vi "DAQ@AddDAQ__Parameter.vi"(1 "ParamterIn":string) -> (0 "ParamterOut":string)   [LabVIEW 2020]
uses:
  MainFrame/Global.vi
panel:
  out "Example Setting:":string
  in  "Dev=":string(combo)
  in  "INTYPE=":string(combo)
  in  "Vmin=":string(combo)
  in  "Vmax=":string(combo)
  in  "Len=":string(combo)
  in  "SPS=":string(combo)
  in  "Ch=":string(combo)
  in  "Driver":string(combo)
  in  "DAQName":string(combo)
  in  "Confirm":bool
  # "Name"
  # "Driver"
  # "Device"
  # "Channel"
  # "Samples Per Second"
  # "SPS"
  # "Range"
  # "~"
  # "Data\nLength"
  # "Second"
  # "Type"
  # "$NAME,NIDAQAI,DEV=,CH=0:1,SPS=,RANGE=-5~5,LEN=,INTYPE=\n$NAME,NIDAQAO,DEV=,CH=0:1,SPS=,RANGE=-5~5"
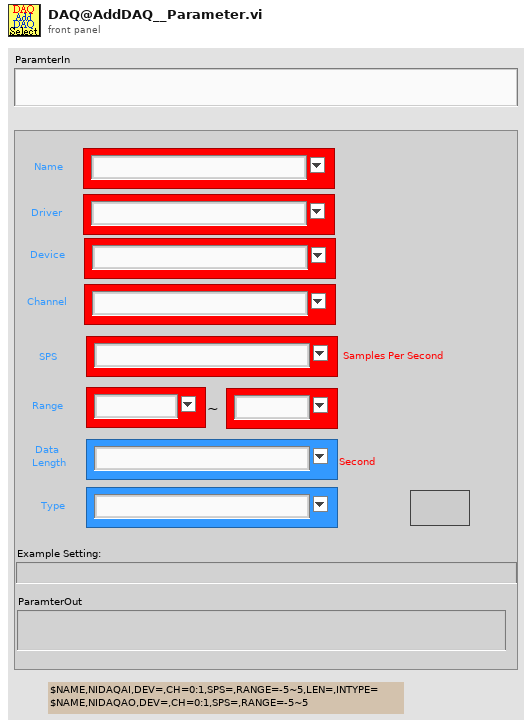
[diagram p1: front panel]
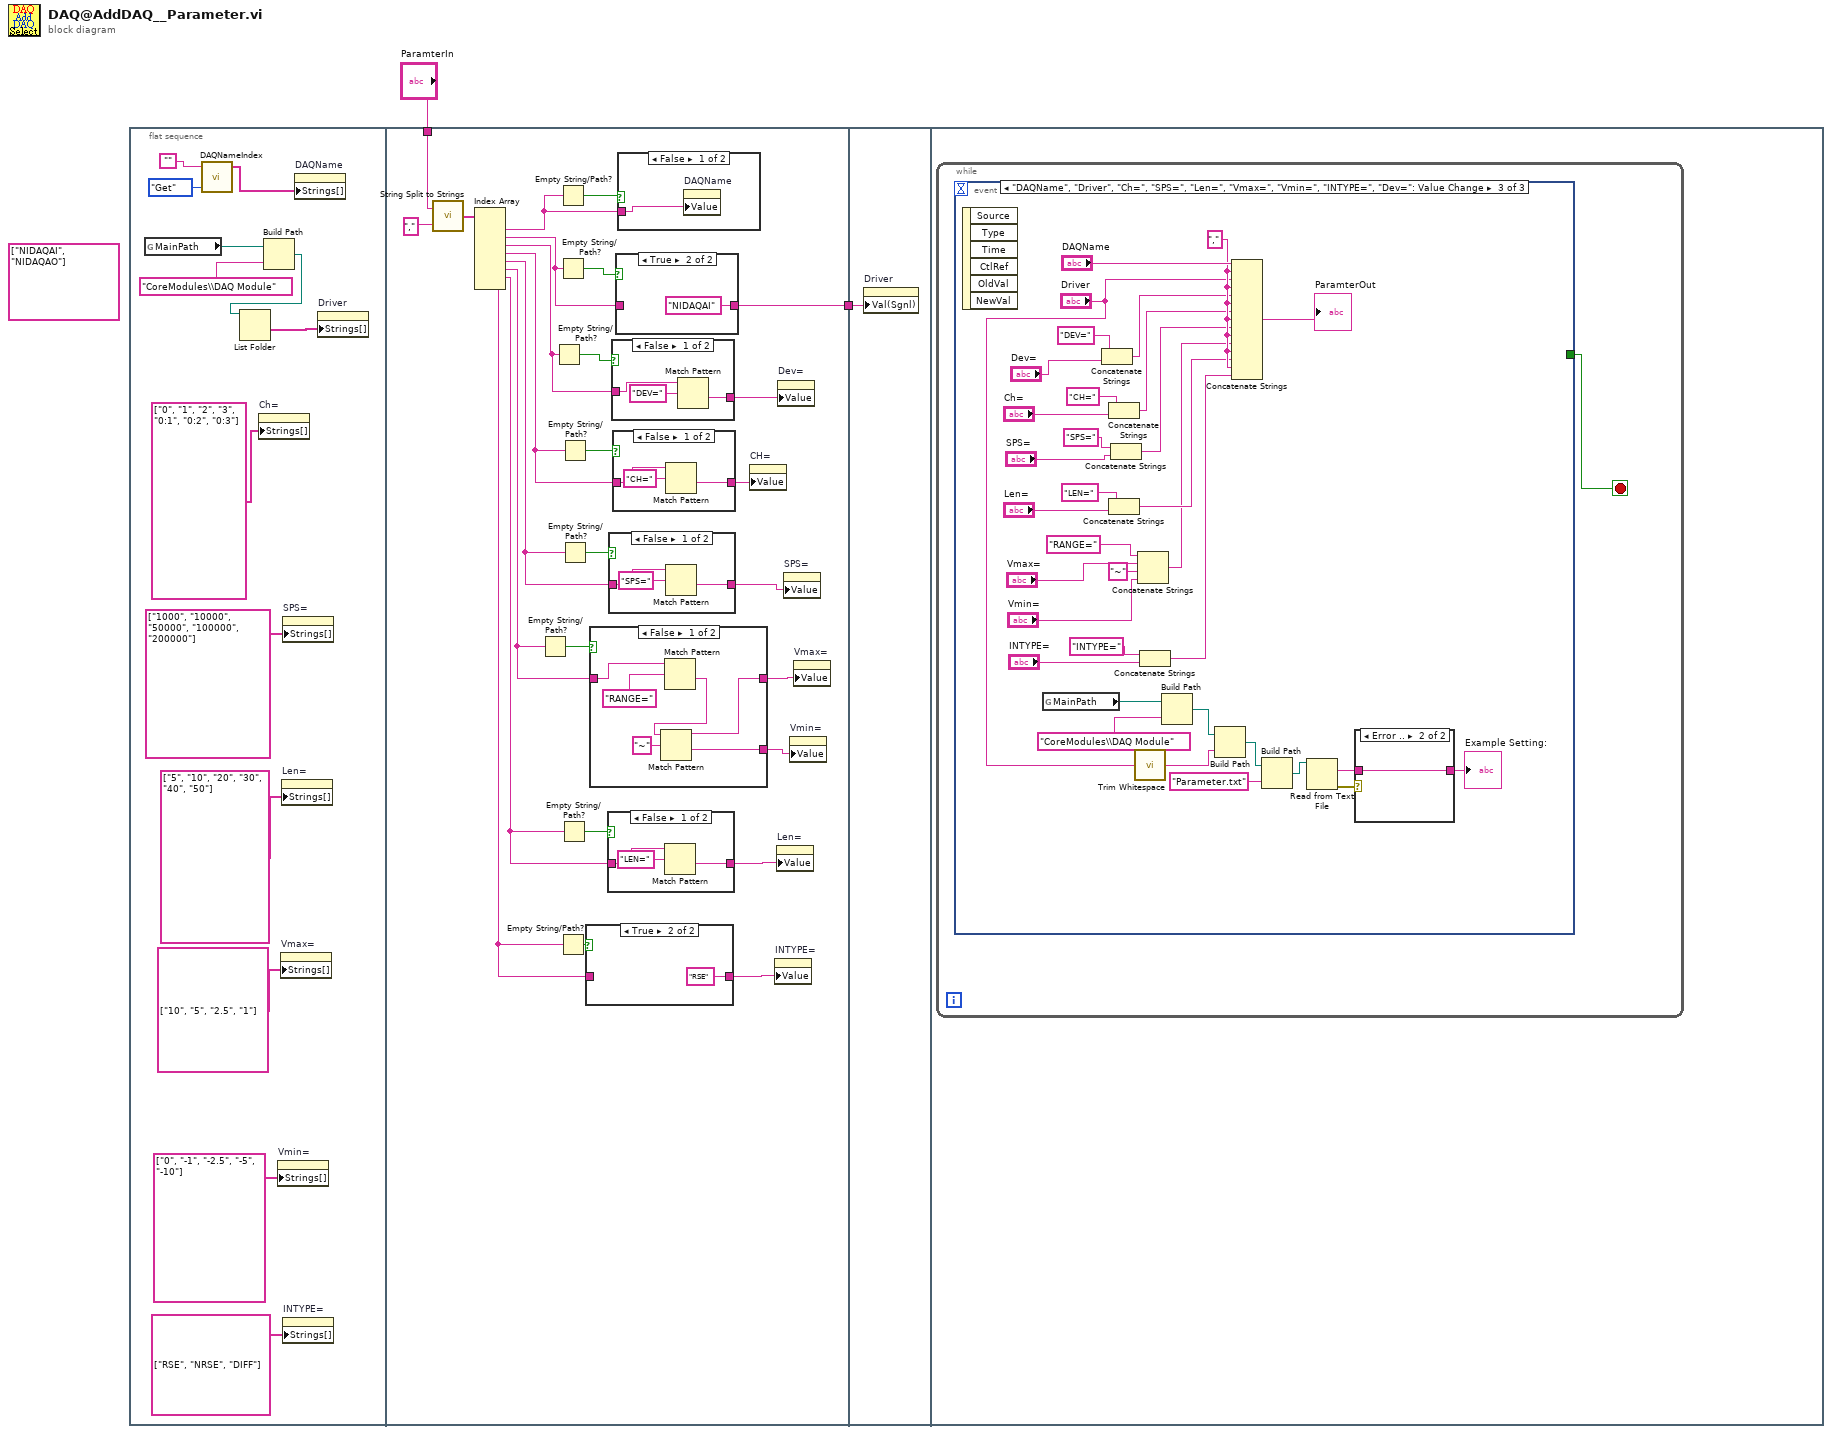
[diagram p0: block diagram]
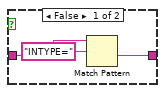
[diagram p3: hidden frame]
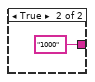
[diagram p4: hidden frame]
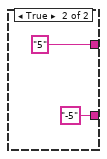
[diagram p5: hidden frame]
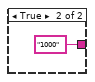
[diagram p6: hidden frame]
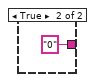
[diagram p7: hidden frame]
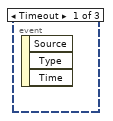
[diagram p10: hidden frame]
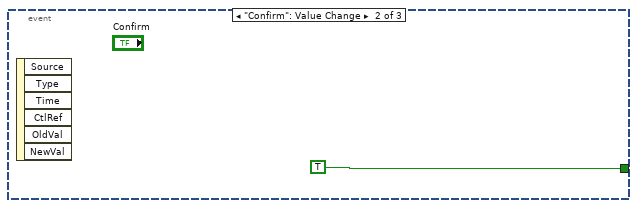
[diagram p11: hidden frame]
diagram:
  (unwired) string[] ["NIDAQAI", "NIDAQAO"] ("Strings []")
  n1 = flat-sequence {
    tunnel: "ParamterIn" -> [w40]
    tunnel: [w33] -> w1
    tunnel: w1 -> [w74]
    frame #0 {
      n2 = global read "Global.vi" "MainPath"() -> (w5:path)
      n3 = call "DAQNameIndex.vi"("OP"=enum16{"Get", "Update", "Init"}."Get", "DAQName"="") -> ("DAQList"=w13:string[])  [unwired: 1 in, 2 out]
      n4 = property on="Ch=" class="CmbBox"("Strings[]"=string[] ["0", "1", "2", "3", "0:1", "0:2", "0:3"] ("Strings []")) -> ()  [unwired: 2 in, 2 out]
      n5 = Build Path(base path=w5, name or relative path="CoreModules\\DAQ Module") -> (appended path=w6:path)
      n6 = List Folder(path=w6) -> (folder names=w3:string[])  [unwired: 3 in, 3 out]
      n7 = property on="Vmin=" class="CmbBox"("Strings[]"=string[] ["0", "-1", "-2.5", "-5", "-10"] ("Strings []")) -> ()  [unwired: 2 in, 2 out]
      n8 = property on="Vmax=" class="CmbBox"("Strings[]"=string[] ["10", "5", "2.5", "1"] ("Strings []")) -> ()  [unwired: 2 in, 2 out]
      n9 = property on="Len=" class="CmbBox"("Strings[]"=string[] ["5", "10", "20", "30", "40", "50"] ("Strings []")) -> ()  [unwired: 2 in, 2 out]
      n10 = property on="SPS=" class="CmbBox"("Strings[]"=string[] ["1000", "10000", "50000", "100000", "200000"] ("Strings []")) -> ()  [unwired: 2 in, 2 out]
      n11 = property on="INTYPE=" class="CmbBox"("Strings[]"=string[] ["RSE", "NRSE", "DIFF"] ("Strings []")) -> ()  [unwired: 2 in, 2 out]
      n12 = property on="DAQName" class="CmbBox"("Strings[]"=w13) -> ()  [unwired: 2 in, 2 out]
      n13 = property on="Driver" class="CmbBox"("Strings[]"=w3) -> ()  [unwired: 2 in, 2 out]
    }
    frame #1 {
      n14 = call "String Split to Strings.vi"("search string/char (-)"=",", "String"=w40) -> ("Array"=w42:string[])
      n15 = Index Array(array=w42) -> (element #1=w38:string, element #2=w36:string, element #3=w17:string, element #4=w19:string, element #5=w20:string, element #6=w21:string, element #7=w23:string, element #8=w22:string)  [unwired: 8 in]
      n16 = Empty String/Path?(string/path=w21) -> (empty?=w30:bool)
      n17 = Empty String/Path?(string/path=w17) -> (empty?=w18:bool)
      n18 = Empty String/Path?(string/path=w38) -> (empty?=w39:bool)
      n19 = Empty String/Path?(string/path=w36) -> (empty?=w37:bool)
      n20 = Empty String/Path?(string/path=w22) -> (empty?=w25:bool)
      n21 = Empty String/Path?(string/path=w23) -> (empty?=w27:bool)
      n22 = Empty String/Path?(string/path=w19) -> (empty?=w35:bool)
      n23 = Empty String/Path?(string/path=w20) -> (empty?=w32:bool)
      n24 = case shown="True" w25 {
        tunnel: [w47 "RSE"] -> w24
        tunnel: w22 -> [w49 _]
        frame False {
          n25 = Match Pattern(string=w49, regular expression="INTYPE=") -> (after substring=w47:string)  [unwired: 1 in, 3 out]
        }
        frame True {
        }
      }
      n26 = case shown="False" w30 {
        tunnel: [w56 "5"] -> w29
        tunnel: w21 -> [w60 _]
        tunnel: [w55 "-5"] -> w28
        frame False {
          n27 = Match Pattern(string=w60, regular expression="RANGE=") -> (after substring=w58:string)  [unwired: 1 in, 3 out]
          n28 = Match Pattern(string=w58, regular expression="~") -> (before substring=w56:string, after substring=w55:string)  [unwired: 1 in, 2 out]
        }
        frame True {
        }
      }
      n29 = case shown="False" w27 {
        tunnel: [w51 "1000"] -> w26
        tunnel: w23 -> [w53 _]
        frame False {
          n30 = Match Pattern(string=w53, regular expression="LEN=") -> (after substring=w51:string)  [unwired: 1 in, 3 out]
        }
        frame True {
        }
      }
      n31 = case shown="False" w32 {
        tunnel: [w63 "1000"] -> w31
        tunnel: w20 -> [w65 _]
        frame False {
          n32 = Match Pattern(string=w65, regular expression="SPS=") -> (after substring=w63:string)  [unwired: 1 in, 3 out]
        }
        frame True {
        }
      }
      n33 = case shown="False" w18 {
        tunnel: w17 -> [w44 w46]
        tunnel: [w43 w46] -> w16
        frame False {
          n34 = Match Pattern(string=w44, regular expression="DEV=") -> (after substring=w43:string)  [unwired: 1 in, 3 out]
        }
        frame True {
        }
      }
      n35 = case shown="False" w35 {
        tunnel: [w67 "0"] -> w34
        tunnel: w19 -> [w69 _]
        frame False {
          n36 = Match Pattern(string=w69, regular expression="CH=") -> (after substring=w67:string)  [unwired: 1 in, 3 out]
        }
        frame True {
        }
      }
      n37 = case shown="True" w37 {
        tunnel: [w71 "NIDAQAI"] -> w33
        tunnel: w36 -> [w71 _]
        frame False {
        }
        frame True {
        }
      }
      n38 = case shown="False" w39 {
        tunnel: w38 -> [w73 _]
        frame False {
          n39 = property on="DAQName" class="CmbBox"("Value"=w73) -> ()  [unwired: 2 in, 2 out]
        }
        frame True {
        }
      }
      n40 = property on="CH=" class="CmbBox"("Value"=w34) -> ()  [unwired: 2 in, 2 out]
      n41 = property on="INTYPE=" class="CmbBox"("Value"=w24) -> ()  [unwired: 2 in, 2 out]
      n42 = property on="Len=" class="CmbBox"("Value"=w26) -> ()  [unwired: 2 in, 2 out]
      n43 = property on="Dev=" class="CmbBox"("Value"=w16) -> ()  [unwired: 2 in, 2 out]
      n44 = property on="SPS=" class="CmbBox"("Value"=w31) -> ()  [unwired: 2 in, 2 out]
      n45 = property on="Vmin=" class="CmbBox"("Value"=w28) -> ()  [unwired: 2 in, 2 out]
      n46 = property on="Vmax=" class="CmbBox"("Value"=w29) -> ()  [unwired: 2 in, 2 out]
    }
    frame #2 {
      n47 = property on="Driver" class="CmbBox"("Val(Sgnl)"=w74) -> ()  [unwired: 2 in, 2 out]
    }
    frame #3 {
      n48 = while {
        stop <- w75 stop-if-true
        n49 = event shown="[2] \"DAQName\", \"Driver\", \"Ch=\", \"SPS=\", \"Len=\", \"Vmax=\", \"Vmin=\", \"INTYPE=\", \"Dev=\": Value Change" {
          selector: _ -> [_ _ _]
          dyn-events: _ -> [_ _ _]
          timeout: _ -> [_ _ _]
          tunnel: [_ TRUE _] -> w75
          event Timeout {
            n50 = event-data() -> ()  [unwired: 1 in, 3 out]
          }
          event "Confirm": Value Change {
            n51 = event-data() -> ()  [unwired: 1 in, 6 out]
          }
          event "DAQName", "Driver", "Ch=", "SPS=", "Len=", "Vmax=", "Vmin=", "INTYPE=", "Dev=": Value Change {
            w93 = "," ("string")
            n52 = event-data() -> ()  [unwired: 1 in, 6 out]
            n53 = global read "Global.vi" "MainPath"() -> (w87:path)
            n54 = Concatenate Strings("DEV=" ("string"), "Dev=") -> (w88:string)
            n55 = Concatenate Strings("CH=" ("string"), "Ch=") -> (w89:string)
            n56 = Concatenate Strings("LEN=" ("string"), "Len=") -> (w92:string)
            n57 = Concatenate Strings("SPS=" ("string"), "SPS=") -> (w90:string)
            n58 = call <vilib>:"Trim Whitespace.vi"("string"="Driver") -> ("trimmed string"=w84:string)  [unwired: 1 in]
            n59 = Concatenate Strings("RANGE=" ("string"), "Vmax=", "~" ("string"), "Vmin=") -> (w91:string)
            n60 = Concatenate Strings("INTYPE=" ("string"), "INTYPE=") -> (w94:string)
            n61 = Build Path(base path=w87, name or relative path="CoreModules\\DAQ Module") -> (appended path=w85:path)
            n62 = Build Path(base path=w85, name or relative path=w84) -> (appended path=w82:path)
            n63 = Concatenate Strings("DAQName", w93, "Driver", w93, w88, w93, w89, w93, w90, w93, w91, w93, w92, w93, w94) -> (→"ParamterOut":string)
            n64 = Build Path(base path=w82, name or relative path="Parameter.txt") -> (appended path=w80:path)
            n65 = Read from Text File(file (use dialog)=w80) -> (text=w78:string, error out=w79:errorcluster)  [unwired: 3 in, 2 out]
            n66 = case shown="Error .." w79 {
              tunnel: [w111 w112] -> w77
              tunnel: w78 -> [w111 w112]
              frame No Error {
              }
              frame Error {
              }
            }
            "Example Setting:" <- w77
          }
        }
      }
    }
  }
